vi "UDP Refresh Last Update Channel.vi"(8 "error in (no error)":errorcluster, 10 "UDP UI References in":T2, 11 "node References":T1) -> (0 "error out":errorcluster, 2 "UDP UI References out":T2, 3 "node References out":T1)   [LabVIEW 2015, in "E2E Tag Exchange editor node.lvclass"]
uses:
  E2E Tag Exchange editor node.lvclass
  implementation specific/UDP/UDP UI References.ctl
  object references.ctl
  <vilib>/NI/DCAF/Tag Editor Core/Configuration Editor/Classes/Engine Parent/Engine Parent Editor Node.lvclass
  <vilib>/NI/Tag Bus/tag/tag descriptor.lvclass/tag descriptor.ctl
  <vilib>/NI/Tag Bus/tag/tag descriptor.lvclass
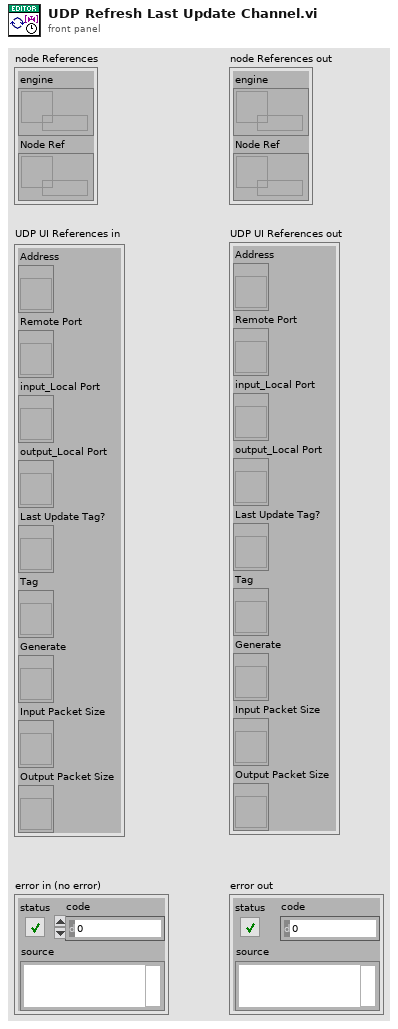
[diagram p1: front panel]
types:
  T1 = typedef "E2E Tag Exchange editor node.lvclass/object references.ctl" = cluster{"engine":refnum<data-value>, "Node Ref":refnum<data-value>}
  T2 = typedef "E2E Tag Exchange editor node.lvclass/UDP UI References.ctl" = cluster{"Address":refnum<vi>, "Remote Port":refnum<vi>, "input_Local Port":refnum<vi>, "output_Local Port":refnum<vi>, "Last Update Tag?":refnum<vi>, "Tag":refnum<vi>, "Generate":refnum<vi>, "Input Packet Size":refnum<vi>, "Output Packet Size":refnum<vi>}
  T3 = enum8{"Enabled", "Disabled", "Disabled and Grayed Out"}
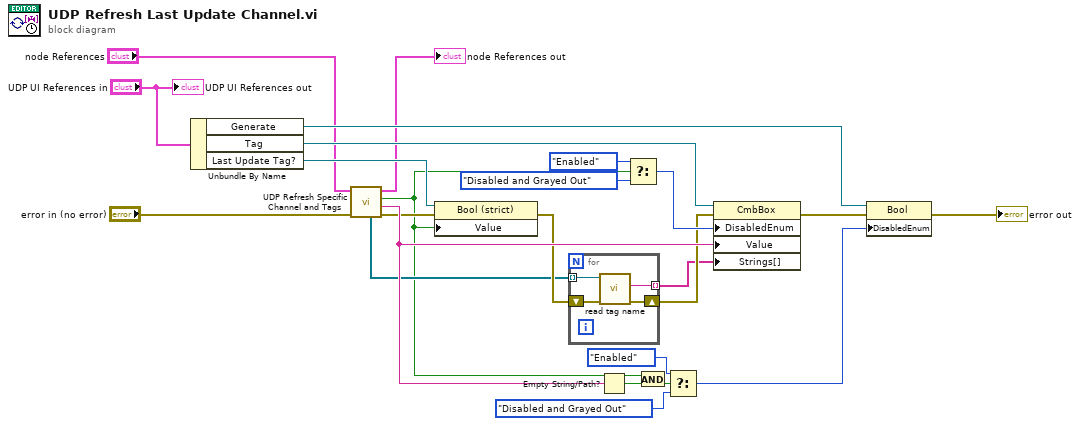
[diagram p0: block diagram]
diagram:
  n1 = Unbundle By Name("UDP UI References in") -> ("Generate"=w18:refnum<vi>, "Tag"=w8:refnum<vi>, "Last Update Tag?"=w7:refnum<vi>)
  n2 = call "UDP Refresh Specific Channel and Tags.vi"("error in (no error)"="error in (no error)", "node References"="node References") -> ("error out"=w6:errorcluster, "Mapped Tag Name"=w16:string, "Channel Exists?"=w1:bool, "node References out"=→"node References out":T1, "tags available for mapping"=w9:refnum<class "tag descriptor.lvclass">[])  [unwired: 5 in]
  n3 = property class="Bool (strict)"(reference=w7, error in=w6, "Value"=w1) -> (error out=w10:errorcluster)  [unwired: 1 out]
  n4 = for {
    tunnel: w9 -> [w28] mode=indexing
    shift-right: [w26] -> w12
    shift-left: w10 -> [w27]
    tunnel: [w25] -> w11 mode=indexing
    n5 = call <vilib>:"read tag name.vi"("error in"=w27, "system tag in"=w28) -> ("error out"=w26:errorcluster, "name"=w25:string)  [unwired: 7 in, 1 out]
  }
  n6 = Empty String/Path?(string/path=w16) -> (empty?=w20:bool)
  n7 = Select(t=T3."Enabled" ("Disabled"), s=w1, f=T3."Disabled and Grayed Out") -> (s? t:f=w15:T3)
  n8 = And(x=w1, y=w20) -> (x .and. y?=w2:bool)
  n9 = Select(t=T3."Enabled" ("Disabled"), s=w2, f=T3."Disabled and Grayed Out") -> (s? t:f=w23:T3)
  n10 = property class="CmbBox"(reference=w8, error in=w12, "DisabledEnum"=w15, "Value"=w16, "Strings[]"=w11) -> (error out=w17:errorcluster)  [unwired: 1 out]
  n11 = property class="Bool"(reference=w18, error in=w17, "DisabledEnum"=w23) -> (error out=→"error out":errorcluster)  [unwired: 1 out]
  "UDP UI References out" <- "UDP UI References in"
